vi "Add Module to Map.vi"(7 "App Ref":refnum<vi>, 8 "error in":errorcluster, 11 "Library In":refnum<class "Library.lvclass">) -> (0 "error out":errorcluster, 3 "Library Out":refnum<class "Library.lvclass">)   [LabVIEW 2019, in "Panther Dashboard.lvlib" / "Library.lvclass"]
uses:
  Library.lvclass
  LabVIEWItem/Item Type--enum.ctl
  Library.lvclass/Library.ctl
  Read Library Ref.vi
  <vilib>/Delacor/Delacor QMH/Libraries/Scripting API/DQMH_Scripting API.lvlib
  LabVIEWItem/LabVIEWItem.lvclass
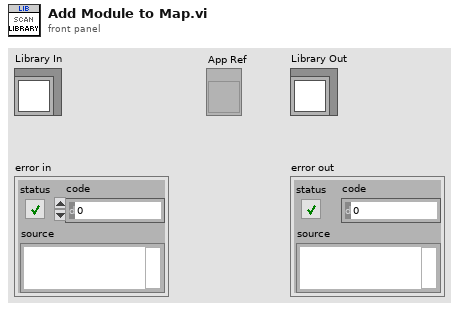
[diagram p1: front panel]
types:
  T1 = typedef "Panther Dashboard.lvlib/LabVIEWItem.lvclass/Item Type--enum.ctl" = enum16{"Requests", "Broadcasts", "Request and Wait for Reply", "Round Trip", "Public API VIs", "» Constant VIs", "» Error VIs", "Module", "Project"}
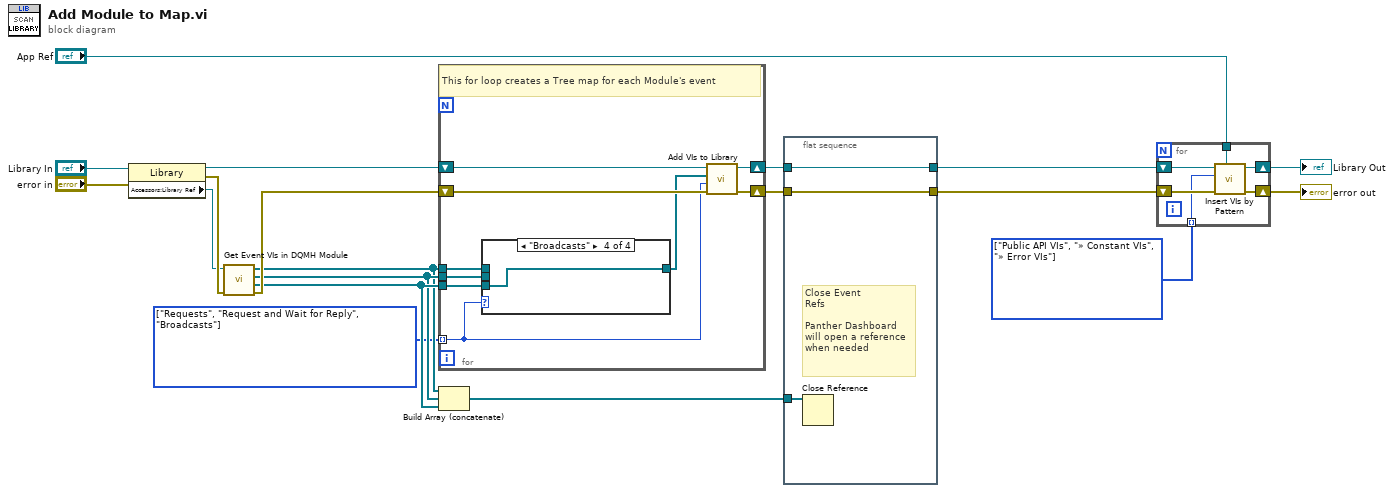
[diagram p0: block diagram]
diagram:
  w1 = T1[] [enum."Public API VIs", enum."» Constant VIs", enum."» Error VIs"] items=["Requests", "Broadcasts", "Request and Wait for Reply", "Round Trip", "Public API VIs", "» Constant VIs", "» Error VIs", "Module", "Project"] ("Array")
  w2 = T1[] [enum."Requests", enum."Request and Wait for Reply", enum."Broadcasts"] items=["Requests", "Broadcasts", "Request and Wait for Reply", "Round Trip", "Public API VIs", "» Constant VIs", "» Error VIs", "Module", "Project"] ("Array")
  n1 = property class="Library"(reference="Library In", error in="error in") -> (reference out=w10:refnum<class "Library.lvclass">, error out=w19:errorcluster, "Accessors:Library Ref"=w9:refnum<vi>)
  n2 = call <vilib>:"Get Event VIs in DQMH Module.vi"("error in"=w19, "DQMH Module"=w9) -> ("error out"=w18:errorcluster, "Broadcast Event VIs"=w7:refnum<vi>[], "Request and Wait for Reply Event VIs"=w6:refnum<vi>[], "Request Event VIs"=w5:refnum<vi>[])  [unwired: 6 in]
  n3 = for {
    tunnel: w2 -> [w21] mode=indexing
    tunnel: w5 -> [w26]
    tunnel: w6 -> [w24]
    tunnel: w7 -> [w25]
    shift-right: [w22] -> w4
    shift-left: w10 -> [w23]
    shift-right: [w27] -> w16
    shift-left: w18 -> [w28]
    # "This for loop creates a Tree map for each Module's event"
    n4 = case shown="\"Broadcasts\"" w21 {
      tunnel: w26 -> [w29 _ _ _]
      tunnel: w25 -> [_ _ _ w31]
      tunnel: w24 -> [_ _ w30 _]
      tunnel: [w29 _ w30 w31] -> w20
      frame "Requests" {
      }
      frame Default {
      }
      frame "Request and Wait for Reply" {
      }
      frame "Broadcasts" {
      }
    }
    n5 = call "Add VIs to Library.vi"("error in"=w28, "Event Type"=w21, "Event VIs"=w20, "Library In"=w23) -> ("error out"=w27:errorcluster, "Library Out"=w22:refnum<class "Library.lvclass">)  [unwired: 6 in]
  }
  n6 = Build Array (concatenate)(w5, w6, w7) -> (w8:refnum<vi>[])
  n7 = flat-sequence {
    tunnel: w8 -> [w33]
    tunnel: w4 -> [w32]
    tunnel: [w32] -> w3
    tunnel: w16 -> [w34]
    tunnel: [w34] -> w15
    frame #0 {
      # "Close Event\nRefs\n\nPanther Dashboard\nwill open a reference\nwhen needed"
      n8 = Close Reference(reference=w33) -> ()  [unwired: 1 in, 1 out]
    }
  }
  n9 = for {
    tunnel: "App Ref" -> [w38]
    shift-right: [w37] -> w11
    shift-left: w3 -> [w36]
    shift-right: [w39] -> w14
    shift-left: w15 -> [w40]
    tunnel: w1 -> [w35] mode=indexing
    n10 = call "Insert VIs by Pattern.vi"("Application in"=w38, "error in"=w40, "VI Type"=w35, "Library In"=w36) -> ("error out"=w39:errorcluster, "Library Out"=w37:refnum<class "Library.lvclass">)  [unwired: 6 in]
  }
  "Library Out" <- w11
  "error out" <- w14
